vi "Debounce Digital Signal.vi"(10 "cycles to filter (0)":u16, 11 "FPGA digital input":refnum<k21>="Port0/DIO0") -> (3 "filtered output":bool)   [LabVIEW 2017, in "NI_Robotics_FPGA Utilities.lvlib"]
uses:
  <vilib>/robotics/Utilities/FPGA Utilities/NI_Robotics_FPGA Utilities.lvlib
  <vilib>/robotics/Utilities/NI_Robotics Utilities.lvlib
  <vilib>/eio/EIONode/EIONode.xnode
  <vilib>/rvi/eio/common/nirviEmuTemplateMethod_errors.vi
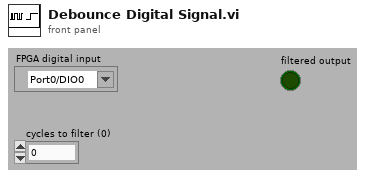
[diagram p1: front panel]
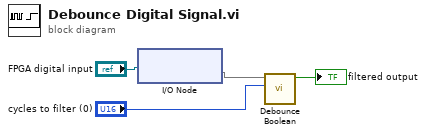
[diagram p0: block diagram]
diagram:
  n1 = xnode "I/O Node"("FPGA I/O In"="FPGA digital input") -> ("I/O Item"=w1)  [unwired: 1 out]
  n2 = call <vilib>:"Debounce Boolean.vi"("cycles to filter (0)"="cycles to filter (0)", "input"=w1) -> ("filtered output"=→"filtered output":bool)  [unwired: 9 in]
